vi "Get All Control References.vi"(5 "Label seulement":bool, 6 "error in (no error)":errorcluster, 7 "In the pane":bool, 8 "Pane refnum":refnum<vi>, 9 "Panel refnum":refnum<vi>) -> (0 "error out":errorcluster, 1 "msec":u32, 2 "Control references [ ]":T1(array[cluster]))   [LabVIEW 2013, in "main.lvlib"]
doc: "The Get All Control References VI recursively determines control references for all objects on the front panel of another VI. This VI takes a front panel reference input and returns an array of references to all controls on that front panel. This VI returns references to all elements of a cluster, including elements in embedded clusters. This VI also returns the element types of arrays embedded in cluster elements.\n\nModifié par Jean-Marc Simard d'Exaprom inc. le 31 août 2009:\n\nAjout des \"Tab Control\" et des contrôles inclus dans les pages des Tab Control. Il est à noter que les références des pages d'un Tab control sont disponibles à travers la référence de ce même Tab Control.\n\nPanel refnum : référence au panel d'un VI\nPane refnum : référence au pane\nIn the pane : les références des contrôles qui sont dans le pane (coin supérieur gauche d'un contrôle incluant le label et le caption - s'ils sont visibles)\nLabel seulement : T - seulement le label apparaît dans la liste des références\n F - le chemin complet d'un contrôle auquel est associée une référence\nControl references [ ] : Liste des références\n Nom : nom (label) du contrôle\n Label?: Label visible ou non\n Caption? Caption visible ou non\n Ref : référence à un contrôle\n\nPar exemple, si un array (Array 1 [ ]) de double (Numérique1) est inclus dans un cluster (Cluster1) alors, nous obtiendrons trois références.\n\nLabel seulement = T\n1) nom = \"Cluster 1\" et sa référence;\n2) nom = \"Array 1\" et la référence à Array 1 [ ];\n3) nom = \"Numérique 1\" et la référence associée à Numérique 1.\n\nLabel seulement = F\n1) nom = \"Cluster 1\" et sa référence;\n2) nom = \"Cluster 1&Array 1\" et la référence à Array 1 [ ];\n3) nom = \"Cluster 1&Array 1 [ ]&Numérique 1\" et la référence associée à Numérique 1."
uses:
  main.lvlib
  <vilib>/Utility/miscctls.llb/LVRectTypeDef.ctl
  <vilib>/Utility/error.llb/DialogType.ctl
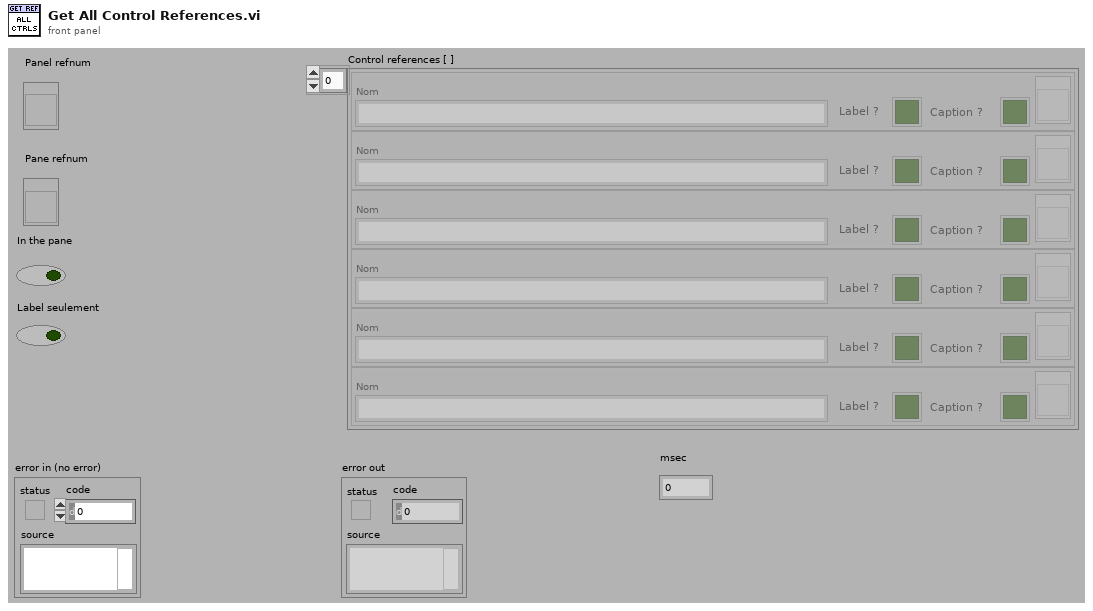
[diagram p1: front panel]
types:
  T1 = cluster{"Nom":string, "Label ?":bool, "Caption ?":bool, "Ref":refnum<vi>}[]
  T2 = typedef "LVRectTypeDef.ctl" = cluster{"Left":i16, "Top":i16, "Right":i16, "Bottom":i16}
  T3 = cluster{"Nom":string, "Label ?":bool, "Caption ?":bool, "Ref":refnum<vi>}
  T4 = typedef "LVPointTypeDef.ctl" = cluster{"Horizontal":i16, "Vertical":i16}
  T5 = typedef "DialogType.ctl" = u16
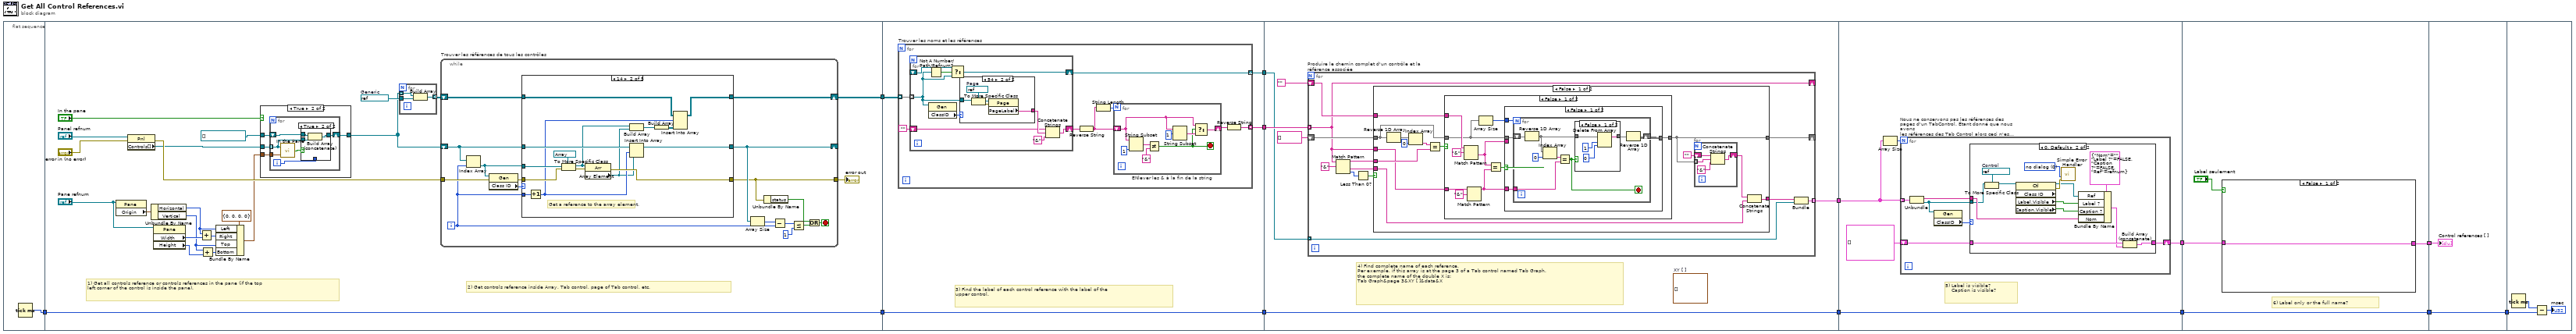
[diagram p0: block diagram]
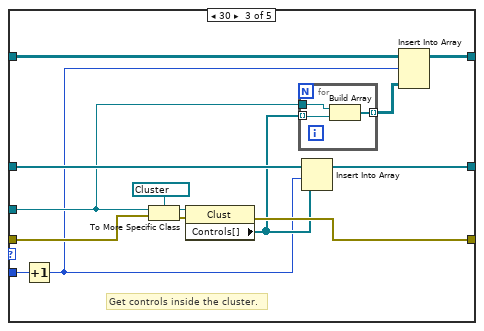
[diagram p5: hidden frame]
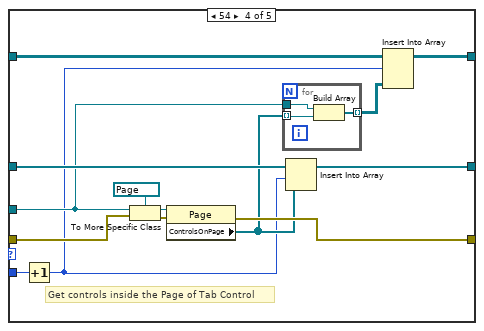
[diagram p6: hidden frame]
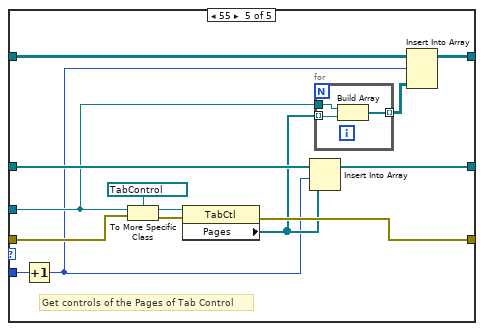
[diagram p7: hidden frame]
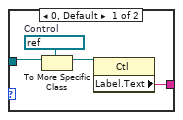
[diagram p8: hidden frame]
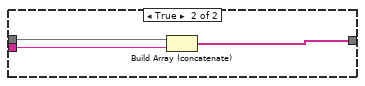
[diagram p10: hidden frame]
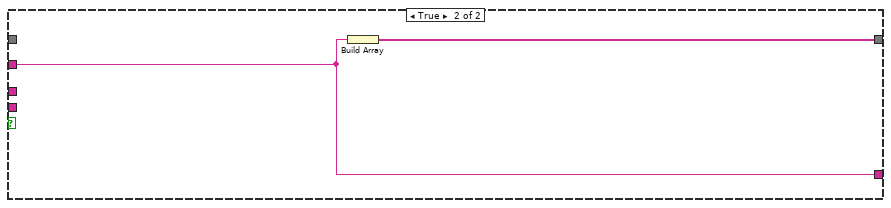
[diagram p12: hidden frame]
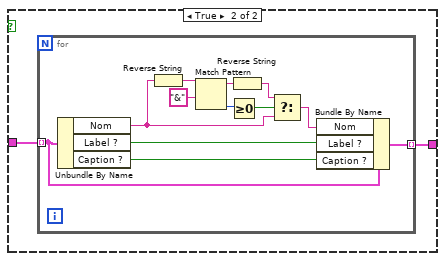
[diagram p14: hidden frame]
diagram:
  n1 = flat-sequence {
    tunnel: [w14] -> w1
    tunnel: [w31] -> w3
    tunnel: [w29] -> w2
    tunnel: w1 -> [w29]
    tunnel: w3 -> [w143]
    tunnel: [w142] -> w13
    tunnel: [w141] -> w12
    tunnel: [w140] -> w4
    tunnel: w2 -> [w140]
    tunnel: w13 -> [w180]
    tunnel: w12 -> [w181]
    tunnel: [w179] -> w11
    tunnel: [w178] -> w5
    tunnel: w4 -> [w178]
    tunnel: w11 -> [w248]
    tunnel: [w247] -> w10
    tunnel: [w246] -> w6
    tunnel: w5 -> [w246]
    tunnel: w10 -> [w274]
    tunnel: [w273] -> w9
    tunnel: [w271] -> w7
    tunnel: w6 -> [w271]
    tunnel: w9 -> [w290]
    tunnel: [w291] -> w8
    tunnel: w7 -> [w291]
    tunnel: w8 -> [w293]
    frame #0 {
      n2 = Tick Count (ms)() -> (millisecond timer value=w14:u32)
    }
    frame #1 {
      w33 = refnum<vi> refnum  # Generic
      # "2) Get controls reference inside Array, Tab control, page of Tab control, etc."
      # "1) Get all controls reference or controls references in the pane (if the top\nleft corner of the control is inside the pane)."
      n3 = property class="Pane"(reference="Pane refnum") -> ("Origin"=w22:T4)  [unwired: 1 in, 2 out]
      n4 = property class="Pnl"(reference="Panel refnum", error in="error in (no error)") -> (error out=w35:errorcluster, "Controls[]"=w15:refnum<vi>[])  [unwired: 1 out]
      n5 = Unbundle By Name(w22) -> ("Horizontal"=w21:i16, "Vertical"=w20:i16)
      n6 = property class="Pane"(reference="Pane refnum") -> ("Width"=w27:u32, "Height"=w25:u32)  [unwired: 1 in, 2 out]
      n7 = Add(x=w21, y=w27) -> (x+y=w26:u32)
      n8 = Add(x=w20, y=w25) -> (x+y=w24:u32)
      n9 = Bundle By Name(cluster=T2 {"Left"=0, "Top"=0, "Right"=0, "Bottom"=0} ("Panel Bounds"), "Left"=w21, "Right"=w26, "Top"=w20, "Bottom"=w24) -> (w19:T2)
      n10 = case shown="True" "In the pane" {
        tunnel: w15 -> [w37 w41]
        tunnel: w19 -> [_ w40]
        tunnel: [w37 w39] -> w18
        tunnel: refnum<vi>[] [] -> [_ w38]
        frame False {
        }
        frame True {
          n11 = for {
            tunnel: w41 -> [w45] mode=indexing
            tunnel: w40 -> [w47]
            shift-right: [w44] -> w39
            shift-left: w38 -> [w43]
            i -> [w42]
            n12 = call "In the Pane.vi"("Panel Bounds"=w47, "Reference"=w45) -> ("Dans le Pane"=w46:bool)
            n13 = case shown="True" w46 {
              tunnel: w45 -> [_ w51]
              tunnel: [w48 w50] -> w44
              tunnel: w43 -> [w48 w49]
              tunnel: w42 -> [_ _]
              frame False {
              }
              frame True {
                n14 = Build Array (concatenate)(w49, w51) -> (w50:refnum<vi>[])
              }
            }
          }
        }
      }
      n15 = for {
        tunnel: w33 -> [w53]
        tunnel: w18 -> [w54] mode=indexing
        tunnel: [w52] -> w32 mode=indexing
        n16 = Build Array(w54, w53) -> (w52:refnum<vi>[])
      }
      n17 = while "Trouver les références de tous les contrôles" {
        shift-right: [w63] -> _
        shift-left: w18 -> [w58]
        tunnel: w35 -> [w62]
        tunnel: [w59] -> w34
        shift-right: [w56] -> w31
        shift-left: w32 -> [w57]
        i -> [w55]
        stop <- w66 stop-if-true
        n18 = Index Array(array=w58, index=w55) -> (element=w64:refnum<vi>)
        n19 = property class="Gen"(reference=w64, error in=w62) -> (error out=w61:errorcluster, "Class ID"=w65:u32)  [unwired: 1 out]
        n20 = case shown="14" w65 {
          tunnel: w64 -> [_ w88 w94 w111 w128]
          tunnel: w58 -> [w73 w87 w101 w118 w135]
          tunnel: w55 -> [_ w86 w90 w107 w124]
          tunnel: [w73 w85 w100 w117 w134] -> w63
          tunnel: w61 -> [w72 w84 w99 w116 w133]
          tunnel: [w72 w82 w97 w114 w131] -> w59
          tunnel: w57 -> [w71 w80 w96 w113 w130]
          tunnel: [w71 w81 w91 w108 w125] -> w56
          frame 0, Default {
          }
          frame 14 {
            # "Get a reference to the array element."
            n21 = Increment(x=w86) -> (x+1=w79:i32)
            n22 = To More Specific Class(target class=refnum<vi> refnum ("target class array"), reference=w88, error in=w84) -> (specific class reference=w78:refnum<vi>, error out=w83:errorcluster)
            n23 = property class="Arr"(reference=w78, error in=w83) -> (error out=w82:errorcluster, "Array Element"=w77:refnum<vi>)  [unwired: 1 out]
            n24 = Build Array(w78, w77) -> (w76:refnum<vi>[])
            n25 = Insert Into Array(array=w87, index=w79, new element=w77) -> (w85:refnum<vi>[])
            n26 = Build Array(w76) -> (w75:refnum<vi>[][])
            n27 = Insert Into Array(array=w80, index (row)=w79, new element=w75) -> (w81:refnum<vi>[][])  [unwired: 1 in]
          }
          frame 30 {
            # "Get controls inside the cluster."
            n28 = Increment(x=w90) -> (x+1=w93:i32)
            n29 = To More Specific Class(target class=refnum<vi> refnum ("target class cluster"), reference=w94, error in=w99) -> (specific class reference=w102:refnum<vi>, error out=w98:errorcluster)
            n30 = property class="Clust"(reference=w102, error in=w98) -> (error out=w97:errorcluster, "Controls[]"=w95:refnum<vi>[])  [unwired: 1 out]
            n31 = for {
              tunnel: w95 -> [w104] mode=indexing
              tunnel: w94 -> [w105]
              tunnel: [w103] -> w92 mode=indexing
              n32 = Build Array(w105, w104) -> (w103:refnum<vi>[])
            }
            n33 = Insert Into Array(array=w101, index=w93, new element=w95) -> (w100:refnum<vi>[])
            n34 = Insert Into Array(array=w96, index (row)=w93, new element=w92) -> (w91:refnum<vi>[][])  [unwired: 1 in]
          }
          frame 54 {
            # "Get controls inside the Page of Tab Control"
            n35 = Increment(x=w107) -> (x+1=w110:i32)
            n36 = To More Specific Class(target class=refnum<vi> refnum ("target class cluster"), reference=w111, error in=w116) -> (specific class reference=w119:refnum<vi>, error out=w115:errorcluster)
            n37 = property class="Page"(reference=w119, error in=w115) -> (error out=w114:errorcluster, "ControlsOnPage"=w112:refnum<vi>[])  [unwired: 1 out]
            n38 = for {
              tunnel: w112 -> [w121] mode=indexing
              tunnel: w111 -> [w122]
              tunnel: [w120] -> w109 mode=indexing
              n39 = Build Array(w122, w121) -> (w120:refnum<vi>[])
            }
            n40 = Insert Into Array(array=w118, index=w110, new element=w112) -> (w117:refnum<vi>[])
            n41 = Insert Into Array(array=w113, index (row)=w110, new element=w109) -> (w108:refnum<vi>[][])  [unwired: 1 in]
          }
          frame 55 {
            # "Get controls of the Pages of Tab Control"
            n42 = Increment(x=w124) -> (x+1=w127:i32)
            n43 = To More Specific Class(target class=refnum<vi> refnum ("target class cluster"), reference=w128, error in=w133) -> (specific class reference=w136:refnum<vi>, error out=w132:errorcluster)
            n44 = property class="TabCtl"(reference=w136, error in=w132) -> (error out=w131:errorcluster, "Pages"=w129:refnum<vi>[])  [unwired: 1 out]
            n45 = Insert Into Array(array=w135, index=w127, new element=w129) -> (w134:refnum<vi>[])
            n46 = for {
              tunnel: w129 -> [w138] mode=indexing
              tunnel: w128 -> [w139]
              tunnel: [w137] -> w126 mode=indexing
              n47 = Build Array(w139, w138) -> (w137:refnum<vi>[])
            }
            n48 = Insert Into Array(array=w130, index (row)=w127, new element=w126) -> (w125:refnum<vi>[][])  [unwired: 1 in]
          }
        }
        n49 = Array Size(array=w63) -> (size(s)=w70:i32)
        n50 = Unbundle By Name(w59) -> ("status"=w60:bool)
        n51 = Subtract(x=w70, y=w55) -> (x-y=w69:i32)
        n52 = Less Or Equal?(x=w69, y=1) -> (x <= y?=w67:bool)
        n53 = Or(x=w60, y=w67) -> (x .or. y?=w66:bool)
      }
      "error out" <- w34
    }
    frame #2 {
      # "3) Find the label of each control reference with the label of the\nupper control."
      n54 = for "Trouver les noms et les références" {
        tunnel: w143 -> [w151] mode=indexing
        tunnel: [w148] -> w141 mode=indexing
        tunnel: [w144] -> w142 mode=indexing
        n55 = for {
          tunnel: w151 -> [w161] mode=indexing
          shift-right: [w168] -> w149
          shift-left: "" -> [w166]
          shift-right: [w163] -> w144
          shift-left: _ -> [w162]
          n56 = property class="Gen"(reference=w161) -> ("ClassID"=w160:u32)  [unwired: 1 in, 2 out]
          n57 = Not A Number/Path/Refnum?(number/path/refnum=w161) -> (NaN/Path/Refnum?=w164:bool)
          n58 = Select(t=w162, s=w164, f=w161) -> (s? t:f=w163:refnum<vi>)
          n59 = case shown="54" w160 {
            tunnel: [w172 w174] -> w167
            tunnel: w161 -> [w170 w173]
            frame 0, Default {
              w171 = refnum<vi> refnum  # Control
              n60 = To More Specific Class(target class=w171, reference=w170) -> (specific class reference=w169:refnum<vi>)  [unwired: 1 in, 1 out]
              n61 = property class="Ctl"(reference=w169) -> ("Label.Text"=w172:string)  [unwired: 1 in, 2 out]
            }
            frame 54 {
              w177 = refnum<vi> refnum  # Page
              n62 = To More Specific Class(target class=w177, reference=w173) -> (specific class reference=w175:refnum<vi>, error out=w176:errorcluster)  [unwired: 1 in]
              n63 = property class="Page"(reference=w175, error in=w176) -> ("PageLabel"=w174:string)  [unwired: 2 out]
            }
          }
          n64 = Concatenate Strings(w166, w167, "&" ("string")) -> (w168:string)
        }
        n65 = Reverse String(1:w149) -> (0:w146:string)
        n66 = String Length(string=w146) -> (length=w147:i32)
        n67 = for "ENlever les & à la fin de la string" {
          N: w147 -> [_]
          shift-right: [w156] -> w145
          shift-left: w146 -> [w155]
          stop <- w152 stop-if-true
          n68 = String Subset(string=w155, length (rest)=1 ("length (rest)")) -> (substring=w158:string)  [unwired: 1 out]
          n69 = Not Equal?(x=w158, y="&") -> (x != y?=w152:bool)
          n70 = String Subset(string=w155, offset (0)=1) -> (substring=w154:string)  [unwired: 1 out]
          n71 = Select(t=w155, s=w152, f=w154) -> (s? t:f=w156:string)
        }
        n72 = Reverse String(1:w145) -> (0:w148:string)
      }
    }
    frame #3 {
      (unwired) cluster{"X":dbl, "Y":dbl}[] []  # XY [ ]
      # "4) Find complete name of each reference.\nPer exemple, if this array is at the page 3 of a Tab control named Tab Graph,\nthe complete name of the double X is:\nTab Graph&page 3&XY [ ]&data&X"
      n73 = for "Produire le chemin complet d'un contrôle et la référence associée" {
        tunnel: w181 -> [w185] mode=indexing
        shift-right: [w192] -> _
        shift-left: string[] [] -> [w191]
        shift-right: [w185] -> _
        shift-left: "" -> [w189]
        tunnel: w180 -> [w184] mode=indexing
        tunnel: [w186] -> w179 mode=indexing
        n74 = Match Pattern(string=w185, regular expression="&") -> (before substring=w190:string, after substring=w188:string, offset past match=w194:i32)  [unwired: 2 out]
        n75 = Less Than 0?(x=w194) -> (x < 0?=w193:bool)
        n76 = case shown="False" w193 {
          tunnel: [w200 w244] -> w192
          tunnel: w185 -> [w202 w245]
          tunnel: [w196 w245] -> w187
          tunnel: w191 -> [w204 _]
          tunnel: w190 -> [w203 _]
          tunnel: w189 -> [w201 _]
          tunnel: w188 -> [w197 _]
          frame False {
            n77 = Reverse 1D Array(array=w204) -> (reversed array=w208:string[])
            n78 = Index Array(array=w208, index=0) -> (element=w206:string)
            n79 = Equal?(x=w206, y=w203) -> (x = y?=w205:bool)
            n80 = case shown="False" w205 {
              tunnel: [w221 w243] -> w200
              tunnel: w204 -> [w213 w243]
              tunnel: w202 -> [w222 _]
              tunnel: w201 -> [w217 _]
              frame False {
                n81 = Match Pattern(string=w217, regular expression="&") -> (after substring=w216:string)  [unwired: 4 out]
                n82 = Match Pattern(string=w222, regular expression="&") -> (before substring=w215:string)  [unwired: 4 out]
                n83 = Array Size(array=w213) -> (size(s)=w214:i32)
                n84 = Equal?(x=w216, y=w215) -> (x = y?=w219:bool)
                n85 = case shown="False" w219 {
                  tunnel: w213 -> [w225 w242]
                  tunnel: [w223 w241] -> w221
                  tunnel: w216 -> [_ w240]
                  tunnel: w215 -> [w226 _]
                  tunnel: w214 -> [w224 _]
                  frame False {
                    n86 = for {
                      N: w224 -> [_]
                      tunnel: w226 -> [w231]
                      shift-right: [w228] -> w223
                      shift-left: w225 -> [w234]
                      stop <- w227 stop-if-true
                      n87 = Reverse 1D Array(array=w234) -> (reversed array=w230:string[])
                      n88 = Index Array(array=w230, index=0) -> (element=w232:string)
                      n89 = Equal?(x=w232, y=w231) -> (x = y?=w227:bool)
                      n90 = case shown="False" w227 {
                        tunnel: [w235 w239] -> w229
                        tunnel: w230 -> [w236 w239]
                        frame False {
                          n91 = Delete From Array(array=w236, length=1, index=0) -> (array with subset deleted=w235:string[])  [unwired: 1 out]
                        }
                        frame True {
                        }
                      }
                      n92 = Reverse 1D Array(array=w229) -> (reversed array=w228:string[])
                    }
                  }
                  frame True {
                    n93 = Build Array (concatenate)(w242, w240) -> (w241:string[])
                  }
                }
              }
              frame True {
              }
            }
            n94 = for {
              tunnel: w200 -> [w211] mode=indexing
              shift-right: [w209] -> w198
              shift-left: "" -> [w212]
              n95 = Concatenate Strings(w212, w211, "&" ("string")) -> (w209:string)
            }
            n96 = Concatenate Strings(w198, w197) -> (w196:string)
          }
          frame True {
            n97 = Build Array(w245) -> (w244:string[])
          }
        }
        n98 = Bundle(w187, w184) -> (w186:cluster{string, refnum<vi>})  [unwired: 1 out]
      }
    }
    frame #4 {
      # "5) Label is visible?\n    Caption is visible?"
      n99 = Array Size(array=w248) -> (size(s)=w250:i32)
      n100 = for "Nous ne conservons pas les références des pages d'un TabControl. Étant donné que nous avons\nles références des Tab Control alors ceci n'est pas nécessaire." {
        N: w250 -> [_]
        tunnel: w248 -> [w256] mode=indexing
        shift-right: [w254] -> w247
        shift-left: T1 [] ("Control references") -> [w255]
        n101 = Unbundle(w256) -> (w253:string, w252:refnum<vi>)
        n102 = property class="Gen"(reference=w252) -> ("ClassID"=w251:u32)  [unwired: 1 in, 2 out]
        n103 = case shown="0, Default" w251 {
          tunnel: w255 -> [w257 w270]
          tunnel: [w257 w269] -> w254
          tunnel: w253 -> [_ w261]
          tunnel: w252 -> [_ w259]
          frame 54 {
          }
          frame 0, Default {
            w260 = refnum<vi> refnum  # Control
            w267 = T5 0 items=["no dialog", "OK message", "continue or stop message", "OK message + warnings", "continue/stop + warnings"] ("type of dialog (OK msg:1)")
            n104 = To More Specific Class(target class=w260, reference=w259) -> (specific class reference=w258:refnum<vi>)  [unwired: 1 in, 1 out]
            n105 = property class="Ctl" props=["Class ID", "Label", "Visible", "Caption", "Visible"](reference=w258) -> (reference out=w265:refnum<vi>, error out=w268:errorcluster, "Label.Visible"=w264:bool, "Caption.Visible"=w263:bool)  [unwired: 1 in, 1 out]
            n106 = call <vilib>:"Simple Error Handler.vi"("type of dialog (OK msg:1)"=w267, "error in (no error)"=w268) -> ()  [unwired: 8 out]
            n107 = Bundle By Name(cluster=T3 {"Nom"="", "Label ?"=FALSE, "Caption ?"=FALSE, "Ref"=refnum}, "Ref"=w265, "Label ?"=w264, "Caption ?"=w263, "Nom"=w261) -> (w262:T3)
            n108 = Build Array (concatenate)(w270, w262) -> (w269:T1)
          }
        }
      }
    }
    frame #5 {
      # "6) Label only or the full name?"
      n109 = case shown="False" "Label seulement" {
        tunnel: w274 -> [w275 w277]
        tunnel: [w275 w276] -> w273
        frame False {
        }
        frame True {
          n110 = for {
            tunnel: w277 -> [w281] mode=indexing
            tunnel: [w278] -> w276 mode=indexing
            n111 = Unbundle By Name(w281) -> ("Nom"=w285:string, "Label ?"=w279:bool, "Caption ?"=w280:bool)
            n112 = Reverse String(1:w285) -> (0:w289:string)
            n113 = Match Pattern(string=w289, regular expression="&") -> (before substring=w284:string, offset past match=w287:i32)  [unwired: 3 out]
            n114 = Greater Or Equal To 0?(x=w287) -> (x >= 0?=w286:bool)
            n115 = Reverse String(1:w284) -> (0:w283:string)
            n116 = Select(t=w283, s=w286, f=w285) -> (s? t:f=w282:string)
            n117 = Bundle By Name(cluster=w281, "Nom"=w282, "Label ?"=w279, "Caption ?"=w280) -> (w278:T3)
          }
        }
      }
    }
    frame #6 {
      "Control references [ ]" <- w290
    }
    frame #7 {
      n118 = Tick Count (ms)() -> (millisecond timer value=w294:u32)
      n119 = Subtract(x=w294, y=w293) -> (x-y=→"msec":u32)
    }
  }
